vi "calib_cam_launcher_tilt (SubVI).vi"(5 "b":dbl format="%#_13g", 7 "a":dbl=1.0, 11 "x":dbl format="%#_13g") -> (3 "y":dbl)   [LabVIEW 2016]
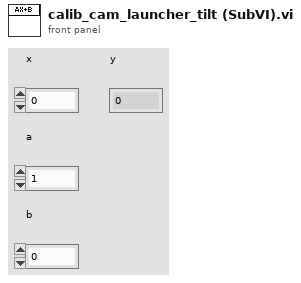
[diagram p1: front panel]
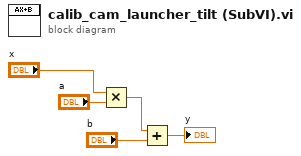
[diagram p0: block diagram]
diagram:
  n1 = Multiply(x="x", y="a") -> (x*y=w1:dbl)
  n2 = Add(x=w1, y="b") -> (x+y=→"y":dbl)
